vi "AlliGator Load Single Gate Image from PTU File.vi"(6 "Action":T1, 8 "error in (no error)":errorcluster, 10 "File Info":variant, 11 "Gate Index":i32) -> (0 "error out":errorcluster, 1 "Data 2":sgl[][](array[numeric]), 3 "Data 1":sgl[][](array[numeric]))   [LabVIEW 2021, in "AlliGator Files.lvlib"]
doc: "Loads single gate image from a .ptu file."
uses:
  AlliGator Files.lvlib
  HDF5/AlliGator FLI Image Stack Action.ctl
  PicoQuant/PTU/LabVIEW/Extended PicoQuant Data File Information.ctl
  PicoQuant/PTU/LabVIEW/PicoQuant Data File Information.ctl
  PicoQuant/PTU/LabVIEW/PicoQuant File Information.ctl
  PicoQuant/PTU/LabVIEW/PicoQuant Software Information.ctl
  PicoQuant/PTU/LabVIEW/PicoQuant Remote Request Information.ctl
  PicoQuant/PTU/LabVIEW/PicoQuant Hardware Information.ctl
  PicoQuant/PTU/LabVIEW/PicoQuant Input Channels.ctl
  PicoQuant/PTU/LabVIEW/PicoQuant Markers.ctl
  PicoQuant/PTU/LabVIEW/PicoQuant Modules.ctl
  PicoQuant/PTU/LabVIEW/PicoQuant Router Channels.ctl
  PicoQuant/PTU/LabVIEW/PicoQuant Measurement Information.ctl
  PicoQuant/PTU/LabVIEW/PicoQuant Image Information.ctl
  PicoQuant/PTU/LabVIEW/PicoQuant Results Format.ctl
  PicoQuant/PTU/LabVIEW/PicoQuant Measurement Results.ctl
  Globals, Variables, Constants/AlliGator Variables List.ctl
  PicoQuant/PTU/LabVIEW/Bin Photons in Pixels.vi
  PicoQuant/PTU/LabVIEW/Bin Nanotimes in Pixel.vi
  PicoQuant/PTU/LabVIEW/PTU Files.lvlib
  PicoQuant/PicoQuant.lvlib
  Globals, Variables, Constants/AlliGator Globals, Variables & Constants.lvlib
  Time/Time.lvlib
  HDF5/AlliGator HDF5.lvlib
panel:
  out "Time (s)":dbl
  # "see the AlliGator License on the block diagram (Ctrl+E or Window:Show Block Diagram)"
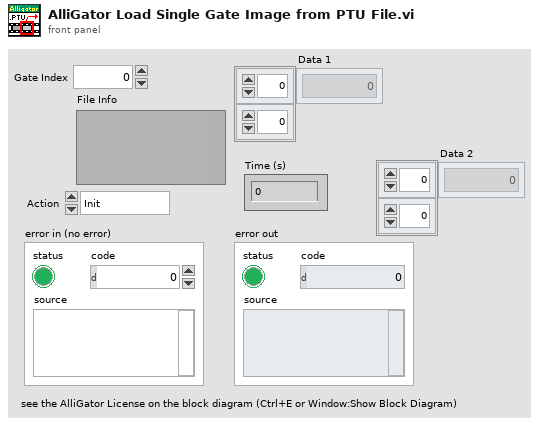
[diagram p1: front panel]
types:
  T1 = typedef "AlliGator HDF5.lvlib/AlliGator FLI Image Stack Action.ctl" = enum16{"Init", "Get Image", "Close"}
  T2 = typedef "PicoQuant.lvlib/Extended PicoQuant Data File Information.ctl" = cluster{"File Path":path, "Data offset (in bytes)":i64, "PicoQuant Data File Information":T3, "User defined # Gates":i64, "User defined Bin Size (s)":dbl, "p (# native bins per user bin)":dbl}
  T3 = typedef "PTU Files.lvlib/PicoQuant Data File Information.ctl" = cluster{"PQ File Information":T4, "PQ Software Information":T5, "PQ Remote Request Information":T6, "PQ Hardware Information":T7, "PQ Measurement Information":T12, "PQ Image Information":T13, "PQ TT Results Format Information":T14, "PQ Measurement Results":T15}
  T4 = typedef "PTU Files.lvlib/PicoQuant File Information.ctl" = cluster{"GUID":string, "Assured Content":string, "Measurement Mode":i64, "Measurement SubMode":i64, "Comment":string, "Creation Time":string}
  T5 = typedef "PTU Files.lvlib/PicoQuant Software Information.ctl" = cluster{"Content Version":string, "Name":string, "Version":string, "# Modules":i64, "Module Names":string[], "Module Versions":string[], "SVN Build":i64}
  T6 = typedef "PTU Files.lvlib/PicoQuant Remote Request Information.ctl" = cluster{"Started by Remote Interface":bool, "Measurement Type":i64, "# Pixel X":i64, "# Pixel Y":i64, "Record Version":i64, "Scanning Pattern":i64, "Scanning Resolution (m/px)":dbl, "Comment":string, "File Name":string, "Group Name":string}
  T7 = typedef "PTU Files.lvlib/PicoQuant Hardware Information.ctl" = cluster{"Input Channels":T8, "Markers":T9, "Modules":T10, "Router Channels":T11}
  T8 = typedef "PTU Files.lvlib/PicoQuant Input Channels.ctl" = cluster{"# Input Channels":i64, "CFD Levels (mV)":i64[], "CFD Zero Crossings (mV)":i64[], "CFD Channel Enabled":bool[], "Module Indices":i64[], "Offsets (ps)":i64[], "Td Codes":i64[], "Trigger Edges":i64[], "Trigger Levels (mV)":i64[]}
  T9 = typedef "PTU Files.lvlib/PicoQuant Markers.ctl" = cluster{"# Markers":i64, "Markers Enabled":bool[], "Holdoff (ns)":i64, "Rising Edges":bool[]}
  T10 = typedef "PTU Files.lvlib/PicoQuant Modules.ctl" = cluster{"# Modules":i64, "Type Codes":i64[], "Version Codes":i64[]}
  T11 = typedef "PTU Files.lvlib/PicoQuant Router Channels.ctl" = cluster{"# Router Channels":i64, "CFD Levels (mV)":i64[], "CFD Present":bool[], "CFD Zero Crossings (mV)":i64[], "Input Levels (mV)":i64[], "Input Types":i64[], "Offsets (ps)":i64[], "Rising Edges":bool[], "Router Enabled":bool, "Router Model Code":i64, "Router Version":string, "Sync CFD Level (mV)":i64, "Sync CFD Zero Crossing (mV)":i64, "Sync Divider":i64, "Sync Offset (ps)":i64, "Sync Trigger Edge":i64, "Sync Trigger Level (mV)":i64, "Trigger Out On":bool, "Trigger Out Period (s)":dbl, "Base Resolution (s)":dbl, "External Devices":i64, "External Reference Clock":bool, "Features":u64, "Part Number":string, "Serial Number (string)":string, "Serial Number":i64, "Timing Mode":i64, "Hardware Type":string, "Hardware Version":string}
  T12 = typedef "PTU Files.lvlib/PicoQuant Measurement Information.ctl" = cluster{"Acquisition Time (ms)":i64, "Binning Factor":i64, "Global Resolution (s)":dbl, "Invalid Sync":bool, "Offset (ns)":u64, "# Curve Parameters":u64, "Devices":string[], "Names":string[], "Start Values":dbl[], "Steps":dbl[], "Stop Values":dbl[], "Tag Names":string[], "Units":string[], "Resolution (s)":dbl, "Restart":bool, "Stop At":u64, "Stop on Over f1":bool}
  T13 = typedef "PTU Files.lvlib/PicoQuant Image Information.ctl" = cluster{"Hardware Acceleration":i64, "Bidirectional":bool, "Dimensions":i64, "Frame Marker":i64, "Scanner Identity":i64, "Learning Time (s)":i64, "Line Frequency":dbl, "Line Start Marker":i64, "Line Stop Marker":i64, "Max Frames":i64, "Objective Name":string, "Pixel Resolution (um)":dbl, "# Pixels X":i64, "# Pixels Y":i64, "Preview Pixels/Line":i64, "Scan Direction":i64, "Sinusoidal Correction":i64, "Time per Line (ms)":dbl, "Time per Pixel (ms)":i64, "Velocity":i64, "X0 (um)":dbl, "X1 (um)":dbl, "X Calibration Offset (V)":dbl, "X Calibration (m/V)":dbl, "Y0 (um)":dbl, "Y1 (um)":dbl, "Y Calibration Offset (V)":dbl, "Y Calibration (m/V)":dbl, "Z0 (um)":dbl, "Z1 (um)":dbl, "Z Calibration Offset (V)":dbl, "Z  Calibration (m/V)":dbl}
  T14 = typedef "PTU Files.lvlib/PicoQuant Results Format.ctl" = cluster{"Bits per Record":i64, "Channel Mask":i64, "Channel Shift ":i64, "DTime Mask":i64, "DTime Shift":i64, "Marker Mask":i64, "Marker Shift":i64, "NSync Mask":i64, "NSync Shift":i64, "Special Mask":i64, "TTTR Record Type":i64, "Wrap Around":i64}
  T15 = typedef "PTU Files.lvlib/PicoQuant Measurement Results.ctl" = cluster{"Stop Reason":i64, "Input Rates (cps)":i64[], "Warning Flags":u64, "# Records":i64, "Stop After (ms)":i64, "Sync Rate (cps)":i64}
  T16 = typedef "AlliGator Globals, Variables & Constants.lvlib/AlliGator Variables List.ctl" = enum16{"---- GUI ----", "GUI:Initialization Status", "GUI:State Indicators Refnum", "GUI:Original AlliGator Menu Items", "GUI:Current Action Loop State", "GUI:Script in progress", "GUI:Playback", "GUI:Loop Playback", "GUI:Search ROI Used", "GUI:Search ROI", "Decay Graph Max Legend Size", "Intensity Graph Max Legend Size", "Decay Statistics Graph Max Legend Size", "Phasor Graph Max Legend Size", "Phasor Ratio Graph Max Legend Size", "Lifetime Graph Max Legend Size", "---- Files ----", "Files:Export Dataset Frames as Individual Files", "Files:Show Batch Export Help Balloons", "Files:Frames in Dataset", "Files:ptu File Frame Start Indices", "Files:Current Frame in Dataset", "Files:Current Frame Timestamp", "Files:Dataset Loaded", "Files:Dataset Metadata", "Files:Dataset Channel", "Files:Dataset Data Description", "Files:Background Dataset Metadata", "Files:Background Dataset Channel", "Files:Background Dataset Data Description", "Files:Background File Subtraction", "Files:Background File Path", "Files:Background File Pile-up Correction", "Files:Background File Pixel Well Capacity", "Files:Background File Scaling Factor", "Files:Current Dataset Load Settings", "Files:Dataset Path", "Files:ICCD-specific Information", "Files:Macrotime Gate Separation", "------ Python Plugins ------", "Python Plugins:Information", "Python Plugins:Python Session", "Python Plugins:Valid Python Session?", "---- Source Image ----", "Source Image:ROIs", "Source Image:Current ROI", "Source Image:ROI Event Refnum", "X_Source Image Display Range", "X_Source Image Palette Information", "X_Type of Displayed Image", "X_Time Gate Slider", "Source Image:Palette List", "Source Image:Scale", "Source Image:ROI Overlay Color", "Source Image:Overlay to Erase", "Source Image:Is Displayed Image Accumulated", "Source Image:White Light Image Modified", "Source Image:Mask Image Modified", "---- Image Profile Window ----", "Image Profile:Window Event Refnum", "Image Profile:IntensityType", "Image Profile:Intensity Average Type", "Image Profile:Intensity-weighted SDV", "Image Profile:Box Profile Type", "Image Profile:Window Open", "Image Profile:Plotted Fit Parameter", "------ Phasor Graph -------", "Phasor Graph:Show Line", "---- Phasor Plot ---", "Phasor Plot:Parameters Changed", "Phasor Plot:FLI Dataset Modified since last Calculation", "Phasor Harmonics Data", "Selected Phasor Harmonics", "Phasor Harmonic Manager Event Refnum", "Phasor Plot:ROIs", "Phasor Plot:Current ROI", "Phasor Plot:ROI Event Refnum", "Phasor Plot:Image Reference Points", "Phasor Plot:Computed", "Phasor Plot:Palette Information", "Phasor Plot:Palette List", "Phasor Plot:Phasor Ratio Palette Information", "Phasor Plot:Phasor Ratio Palette List", "Phasor Plot:Image Scale", "Phasor Plot:Image Overlay to Erase", "Phasor Plot:Image Elements to Update", "Phasor Plot:Current Calculation Parameters", "Phasor Plot:Current Calibration Options", "Phasor Plot:Reset Cumulated Phasor Plot", "Phasor Plot:Reference 1", "Phasor Plot:Lifetime Reference 1", "Phasor Plot:Reference 1 Frequency", "Phasor Plot:Reference 2", "Phasor Plot:Lifetime Reference 2", "Phasor Plot:Reference 2 Frequency", "---- Decay Analysis ----", "Number of Selected Decays to Fit", "LS Fit Results", "LAR Fit Results", "BS Fit Results", "Last Decay Max - Min", "Best Fit Parameters", "Best Fit Parameter Names", "Actual Size X", "Actual Size Y", "Binning X", "Binning Y", "Actual # Gates", "Dataset Number", "Gates to...", "Gates Skipped", "Gates to keep", "Gate Step", "Gate Separation", "Reversed Gates", "Pile-up Correction", "Pixel Well Capacity", "Background Subtracted", "Background Subtraction Method", "Background Definition Range", "Background File (deprecated)", "Number of Dataset Accumulated", "Array of Accumulated Dataset Paths", "Do Averaged Datasets", "Destination File Path", "Process Plot Target", "Use 1/D as Phasor Frequency", "---- Decay Fit Parameter Map -----", "Decay Fit Parameter Map:Palette Information", "Decay Fit Parameter Map:Palette List", "---- Parameter Map ----", "Parameter Map:Palette Information", "Parameter Map:Palette List", "------- Local Decay Window ---------", "Local Decay Graph Window:Event Refnum", "Local Decay Graph Window:Use normalized IRF for convolution", "----- Miscellaneous ----", "Misc:Skippable Dialog Windows Status"}
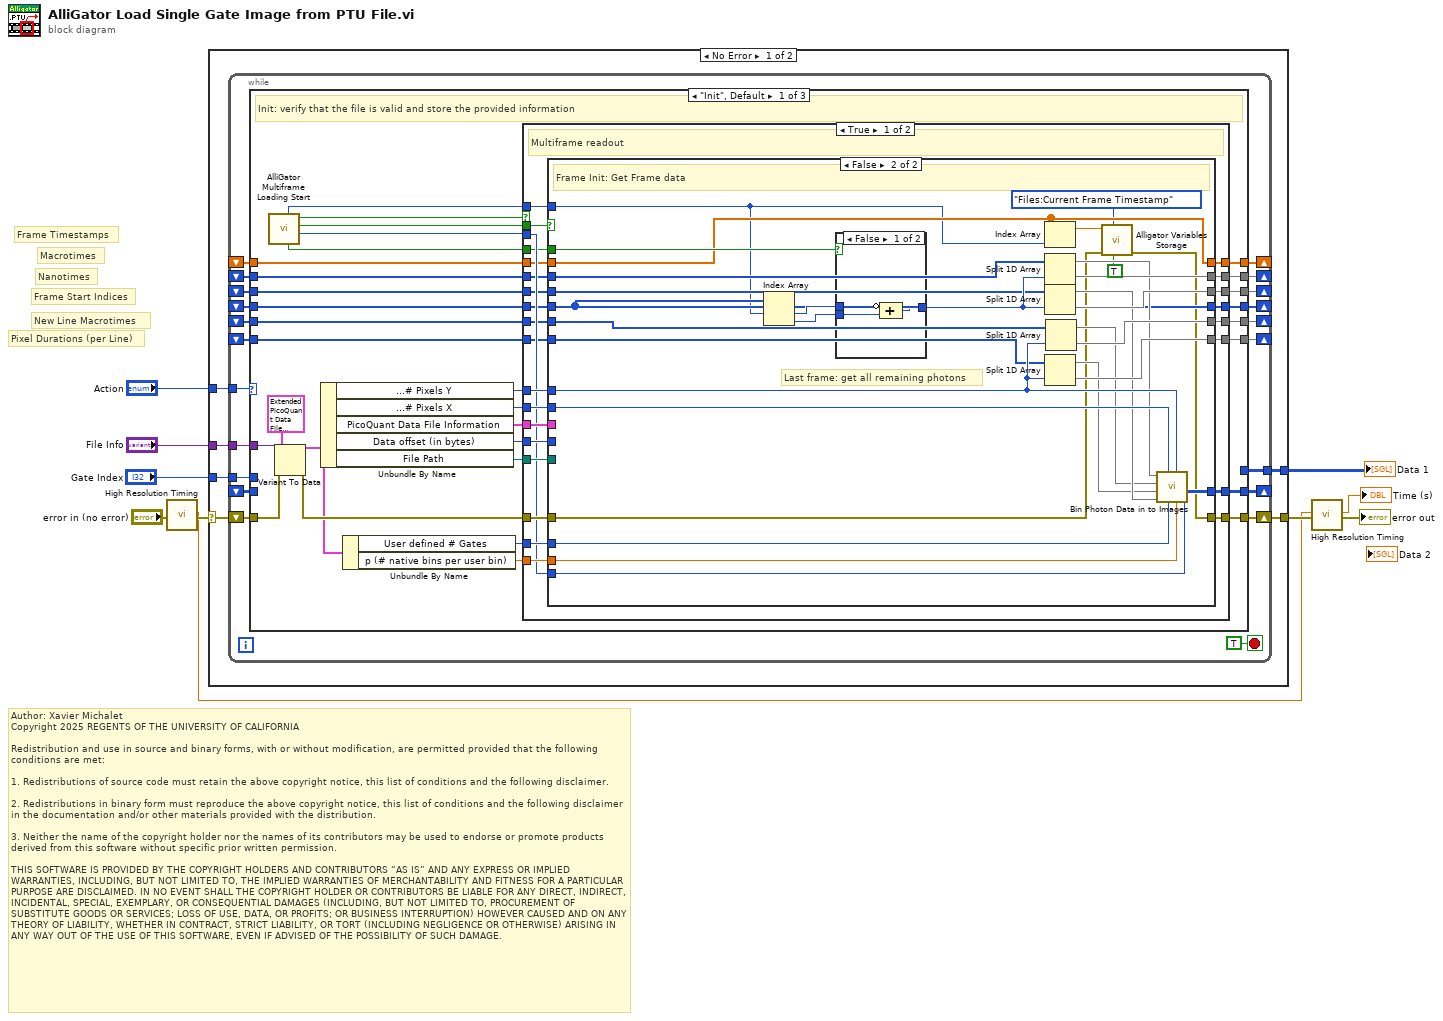
[diagram p0: block diagram]
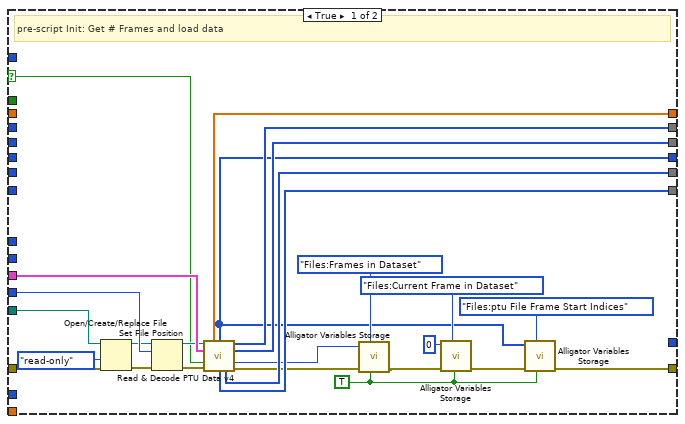
[diagram p2: hidden frame]
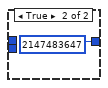
[diagram p3: hidden frame]
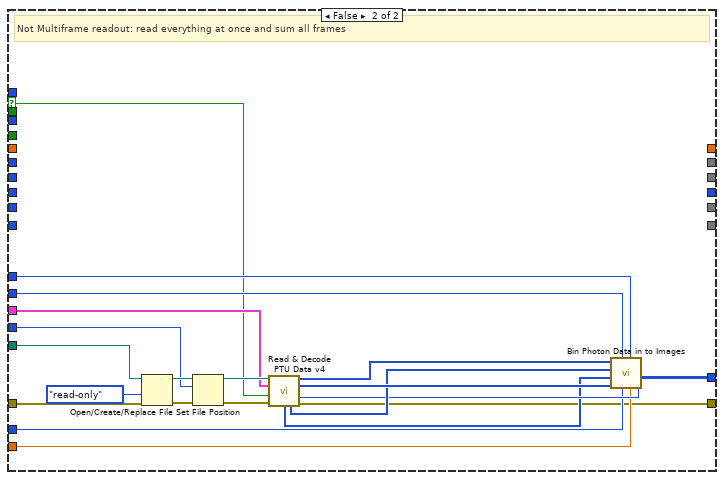
[diagram p4: hidden frame]
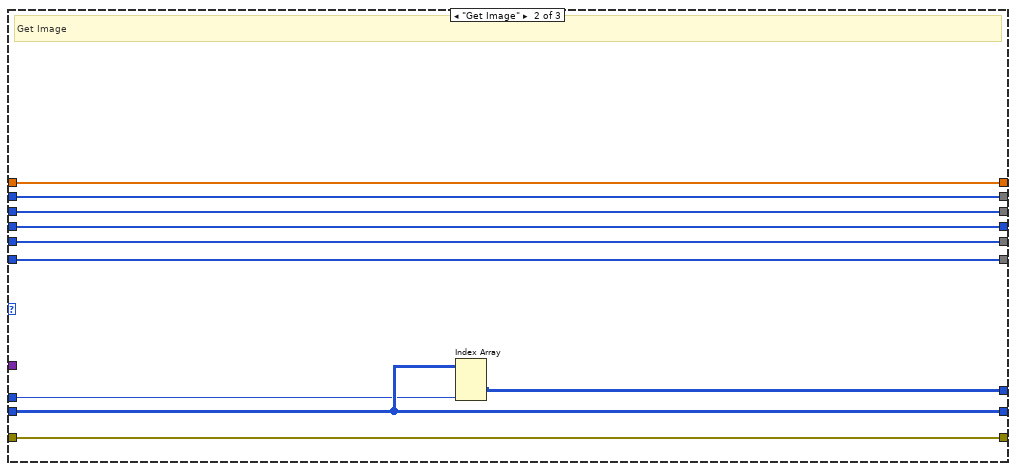
[diagram p5: hidden frame]
diagram:
  # "Author: Xavier Michalet\nCopyright 2025 REGENTS OF THE UNIVERSITY OF CALIFORNIA\n\nRedistribution and use in source and binary forms, with or without modification, are permitted provided that the following conditions are met:\n\n1. Redistributions of source code must retain the above copyright notice, this list of conditions and the following disclaimer.\n\n2. Redistributions in binary form must reproduce the above copyright notice, this list of conditions and the following disclaimer in the documentation and/or other materials provided with the distribution.\n\n3. Neither the name of the copyright holder nor the names of its contributors may be used to endorse or promote products derived from this software without specific prior written permission.\n\nTHIS SOFTWARE IS PROVIDED BY THE COPYRIGHT HOLDERS AND CONTRIBUTORS “AS IS” AND ANY EXPRESS OR IMPLIED WARRANTIES, INCLUDING, BUT NOT LIMITED TO, THE IMPLIED WARRANTIES OF MERCHANTABILITY AND FITNESS FOR A PARTICULAR PURPOSE ARE DISCLAIMED. IN NO EVENT SHALL THE COPYRIGHT HOLDER OR CONTRIBUTORS BE LIABLE FOR ANY DIRECT, INDIRECT, INCIDENTAL, SPECIAL, EXEMPLARY, OR CONSEQUENTIAL DAMAGES (INCLUDING, BUT NOT LIMITED TO, PROCUREMENT OF SUBSTITUTE GOODS OR SERVICES; LOSS OF USE, DATA, OR PROFITS; OR BUSINESS INTERRUPTION) HOWEVER CAUSED AND ON ANY THEORY OF LIABILITY, WHETHER IN CONTRACT, STRICT LIABILITY, OR TORT (INCLUDING NEGLIGENCE OR OTHERWISE) ARISING IN ANY WAY OUT OF THE USE OF THIS SOFTWARE, EVEN IF ADVISED OF THE POSSIBILITY OF SUCH DAMAGE."
  # "Frame Timestamps"
  # "Pixel Durations (per Line)"
  # "New Line Macrotimes"
  # "Nanotimes"
  # "Macrotimes"
  # "Frame Start Indices"
  n1 = call "High Resolution Timing.vi"("Error In"="error in (no error)") -> ("elapsed (relative) seconds"=w2:dbl, "Error Out"=w4:errorcluster)  [unwired: 16 in, 1 out]
  n2 = case shown="No Error" w4 {
    selector: w4 -> [w15 w193]
    tunnel: [w14 w193] -> w9
    tunnel: "Action" -> [w16 _]
    tunnel: "File Info" -> [w13 _]
    tunnel: "Gate Index" -> [w12 _]
    tunnel: [w11 _] -> w5
    frame No Error {
      n3 = while {
        tunnel: w16 -> [w36]
        tunnel: w13 -> [w33]
        tunnel: w12 -> [w32]
        tunnel: [w31] -> w11
        shift-right: [w30] -> _
        shift-left: _ -> [w29]
        shift-right: [w34] -> w14
        shift-left: w15 -> [w35]
        shift-right: [w28] -> _
        shift-left: _ -> [w25]
        shift-right: [w27] -> _
        shift-left: _ -> [w24]
        shift-right: [w26] -> _
        shift-left: _ -> [w23]
        shift-right: [w22] -> _
        shift-left: _ -> [w20]
        shift-right: [w21] -> _
        shift-left: _ -> [w19]
        shift-right: [w18] -> _
        shift-left: _ -> [w17]
        stop <- TRUE stop-if-true
        n4 = case shown="\"Init\", Default" w36 {
          tunnel: w35 -> [w67 w185 w192]
          tunnel: [w40 w185 w192] -> w34
          tunnel: w33 -> [w68 _ _]
          tunnel: w32 -> [_ w183 _]
          tunnel: [_ w182 _] -> w31
          tunnel: [w63 w184 _] -> w30
          tunnel: w29 -> [_ w184 _]
          tunnel: [w62 w181 w191] -> w28
          tunnel: [w61 w180 w190] -> w27
          tunnel: [w60 w179 w189] -> w26
          tunnel: w25 -> [w50 w181 w191]
          tunnel: w24 -> [w49 w180 w190]
          tunnel: w23 -> [w48 w179 w189]
          tunnel: [w47 w178 w188] -> w22
          tunnel: [w46 w177 w187] -> w21
          tunnel: w20 -> [w45 w178 w188]
          tunnel: w19 -> [w44 w177 w187]
          tunnel: [w39 w176 w186] -> w18
          tunnel: w17 -> [w38 w176 w186]
          frame "Init", Default {
            # "Init: verify that the file is valid and store the provided information"
            n5 = call "AlliGator Multiframe Loading Start.vi"() -> ("# Frames"=w43:i32, "Multiframe Start?"=w51:bool, "Multiframe?"=w52:bool, "Last Frame?"=w41:bool, "Current Frame Index"=w42:i32)  [unwired: 6 in, 1 out]
            n6 = Variant To Data(error in=w67, type=T2 {"File Path"=path "", "Data offset (in bytes)"=0, "PicoQuant Data File Information"={"PQ File Information"={"GUID"="", "Assured Content"="", "Measurement Mode"=0, "Measurement SubMode"=0, "Comment"="", "Creation Time"=""}, "PQ Software Information"={"Content Version"="", "Name"="", "Version"="", "# Modules"=0, "Module Names"=[], "Module Versions"=[], "SVN Build"=0}, "PQ Remote Request Information"={"Started by Remote Interface"=FALSE, "Measurement Type"=0, "# Pixel X"=0, "# Pixel Y"=0, "Record Version"=0, "Scanning Pattern"=0, "Scanning Resolution (m/px)"=0.0, "Comment"="", "File Name"="", "Group Name"=""}, "PQ Hardware Information"={"Input Channels"={"# Input Channels"=0, "CFD Levels (mV)"=[], "CFD Zero Crossings (mV)"=[], "CFD Channel Enabled"=[], "Module Indices"=[], "Offsets (ps)"=[], "Td Codes"=[], "Trigger Edges"=[], "Trigger Levels (mV)"=[]}, "Markers"={"# Markers"=0, "Markers Enabled"=[], "Holdoff (ns)"=0, "Rising Edges"=[]}, "Modules"={"# Modules"=0, "Type Codes"=[], "Version Codes"=[]}, "Router Channels"={"# Router Channels"=0, "CFD Levels (mV)"=[], "CFD Present"=[], "CFD Zero Crossings (mV)"=[], "Input Levels (mV)"=[], "Input Types"=[], "Offsets (ps)"=[], "Rising Edges"=[], "Router Enabled"=FALSE, "Router Model Code"=0, "Router Version"="", "Sync CFD Level (mV)"=0, "Sync CFD Zero Crossing (mV)"=0, "Sync Divider"=0, "Sync Offset (ps)"=0, "Sync Trigger Edge"=0, "Sync Trigger Level (mV)"=0, "Trigger Out On"=FALSE, "Trigger Out Period (s)"=0.0, "Base Resolution (s)"=0.0, "External Devices"=0, "External Reference Clock"=FALSE, "Features"=0, "Part Number"="", "Serial Number (string)"="", "Serial Number"=0, "Timing Mode"=0, "Hardware Type"="", "Hardware Version"=""}}, "PQ Measurement Information"={"Acquisition Time (ms)"=0, "Binning Factor"=0, "Global Resolution (s)"=0.0, "Invalid Sync"=FALSE, "Offset (ns)"=0, "# Curve Parameters"=0, "Devices"=[], "Names"=[], "Start Values"=[], "Steps"=[], "Stop Values"=[], "Tag Names"=[], "Units"=[], "Resolution (s)"=0.0, "Restart"=FALSE, "Stop At"=0, "Stop on Over f1"=FALSE}, "PQ Image Information"={"Hardware Acceleration"=0, "Bidirectional"=FALSE, "Dimensions"=0, "Frame Marker"=0, "Scanner Identity"=0, "Learning Time (s)"=0, "Line Frequency"=0.0, "Line Start Marker"=0, "Line Stop Marker"=0, "Max Frames"=0, "Objective Name"="", "Pixel Resolution (um)"=0.0, "# Pixels X"=0, "# Pixels Y"=0, "Preview Pixels/Line"=0, "Scan Direction"=0, "Sinusoidal Correction"=0, "Time per Line (ms)"=0.0, "Time per Pixel (ms)"=0, "Velocity"=0, "X0 (um)"=0.0, "X1 (um)"=0.0, "X Calibration Offset (V)"=0.0, "X Calibration (m/V)"=0.0, "Y0 (um)"=0.0, "Y1 (um)"=0.0, "Y Calibration Offset (V)"=0.0, "Y Calibration (m/V)"=0.0, "Z0 (um)"=0.0, "Z1 (um)"=0.0, "Z Calibration Offset (V)"=0.0, "Z  Calibration (m/V)"=0.0}, "PQ TT Results Format Information"={"Bits per Record"=0, "Channel Mask"=0, "Channel Shift "=0, "DTime Mask"=0, "DTime Shift"=0, "Marker Mask"=0, "Marker Shift"=0, "NSync Mask"=0, "NSync Shift"=0, "Special Mask"=0, "TTTR Record Type"=0, "Wrap Around"=0}, "PQ Measurement Results"={"Stop Reason"=0, "Input Rates (cps)"=[], "Warning Flags"=0, "# Records"=0, "Stop After (ms)"=0, "Sync Rate (cps)"=0}}, "User defined # Gates"=0, "User defined Bin Size (s)"=0.0, "p (# native bins per user bin)"=0.0} ("Extended PicoQuant Data File Information"), Variant=w68) -> (data=w64:T2, error out=w66:errorcluster)
            n7 = Unbundle By Name(w64) -> ("PicoQuant Data File Information.PQ Image Information.# Pixels Y"=w57:i64, "PicoQuant Data File Information.PQ Image Information.# Pixels X"=w56:i64, "PicoQuant Data File Information"=w55:T3, "Data offset (in bytes)"=w59:i64, "File Path"=w58:path)
            n8 = Unbundle By Name(w64) -> ("User defined # Gates"=w54:i64, "p (# native bins per user bin)"=w53:dbl)
            n9 = case shown="True" w52 {
              selector: w52 -> [_ w155]
              tunnel: w66 -> [w94 w175]
              tunnel: [w93 w174] -> w63
              tunnel: [w86 _] -> w62
              tunnel: [w85 _] -> w61
              tunnel: [w81 _] -> w60
              tunnel: w59 -> [w92 w164]
              tunnel: w58 -> [w91 w162]
              tunnel: w57 -> [w84 w161]
              tunnel: w56 -> [w90 w160]
              tunnel: w55 -> [w89 w159]
              tunnel: w54 -> [w88 w158]
              tunnel: w53 -> [w87 w157]
              tunnel: w51 -> [w77 _]
              tunnel: w50 -> [w76 _]
              tunnel: w49 -> [w75 _]
              tunnel: w48 -> [w74 _]
              tunnel: [w83 _] -> w47
              tunnel: [w82 _] -> w46
              tunnel: w43 -> [w80 _]
              tunnel: w45 -> [w73 _]
              tunnel: w44 -> [w72 _]
              tunnel: w42 -> [w79 _]
              tunnel: w41 -> [w78 _]
              tunnel: [w71 w156] -> w40
              tunnel: [w70 _] -> w39
              tunnel: w38 -> [w69 _]
              frame True {
                # "Multiframe readout"
                n10 = case shown="False" w77 {
                  selector: w77 -> [w96 _]
                  tunnel: w94 -> [w120 w122]
                  tunnel: [_ w150] -> w93
                  tunnel: w92 -> [w119 _]
                  tunnel: w91 -> [w118 _]
                  tunnel: w90 -> [_ w149]
                  tunnel: w89 -> [w117 _]
                  tunnel: w88 -> [_ w148]
                  tunnel: w87 -> [_ w147]
                  tunnel: [w111 w146] -> w86
                  tunnel: [w110 w145] -> w85
                  tunnel: w84 -> [_ w144]
                  tunnel: [w109 w143] -> w83
                  tunnel: [w108 w142] -> w82
                  tunnel: [w97 w130] -> w81
                  tunnel: w80 -> [_ w141]
                  tunnel: w79 -> [_ w126]
                  tunnel: w78 -> [_ w140]
                  tunnel: w76 -> [_ w132]
                  tunnel: w75 -> [_ w131]
                  tunnel: w74 -> [_ w130]
                  tunnel: w73 -> [_ w129]
                  tunnel: w72 -> [_ w128]
                  tunnel: [w100 w121] -> w71
                  tunnel: [w95 w127] -> w70
                  tunnel: w69 -> [_ w127]
                  frame True {
                    w99 = TRUE ("Get(F)/Set")
                    # "pre-script Init: Get # Frames and load data"
                    n11 = Open/Create/Replace File(file path (use dialog)=w118, error in=w120, access (0:read/write)=enum16{"read/write", "read-only", "write-only"}."read-only") -> (refnum out=w113:refnum<file>, error out=w116:errorcluster)  [unwired: 3 in, 1 out]
                    n12 = Set File Position(offset (in bytes) (0)=w119, refnum=w113, error in=w116) -> (refnum out=w112:refnum<file>, error out=w114:errorcluster)  [unwired: 1 in]
                    n13 = call "Read & Decode PTU Data v4.vi"("Byte Stream File in"=w112, "PicoQuant Data File Information"=w117, "Multiframe Readout"=w96, "error in (no error)"=w114) -> ("Frame Timestamps (s)"=w95:dbl[], "Frame Start Indices"=w97:i32[], "Macrotimes"=w111:u64[], "Nanotimes"=w110:u32[], "# Frames (inferred)"=w105:i32, "Pixel Durations (inferred_"=w108:i64[], "Line Start Macrotimes"=w109:u64[], "Error Out"=w107:errorcluster)  [unwired: 2 in, 2 out]
                    n14 = call "Alligator Variables Storage.vi"("Get(F)/Set"=w99, "AlliGator Variable"=AlliGator_Variables_List."Files:Frames in Dataset" ("Alligator Variable"), "Error In"=w107, "Data in"=w105) -> ("Error Out"=w104:errorcluster)  [unwired: 5 in, 2 out]
                    n15 = call "Alligator Variables Storage.vi"("Get(F)/Set"=w99, "AlliGator Variable"=AlliGator_Variables_List."Files:Current Frame in Dataset" ("Alligator Variable"), "Error In"=w104, "Data in"=0 ("# Frames")) -> ("Error Out"=w101:errorcluster)  [unwired: 5 in, 2 out]
                    n16 = call "Alligator Variables Storage.vi"("Get(F)/Set"=w99, "AlliGator Variable"=AlliGator_Variables_List."Files:ptu File Frame Start Indices" ("Alligator Variable"), "Error In"=w101, "Data in"=w97) -> ("Error Out"=w100:errorcluster)  [unwired: 5 in, 2 out]
                  }
                  frame False {
                    # "Last frame: get all remaining photons"
                    # "Frame Init: Get Frame data"
                    n17 = Index Array(array=w130, index #1=w126) -> (element #1=w135:i32, element #2=w134:i32)  [unwired: 1 in]
                    n18 = case shown="False" w140 {
                      tunnel: w135 -> [w153 _]
                      tunnel: w134 -> [w152 _]
                      tunnel: [w151 2147483647] -> w133
                      frame False {
                        n19 = Compound Arithmetic op=ADD(invert w153, w152) -> (w151:i32)
                      }
                      frame True {
                      }
                    }
                    n20 = Index Array(array=w127, index=w126) -> (element=w125:dbl)
                    n21 = Split 1D Array(array=w132, index=w133) -> (first subarray=w139:u64[], second subarray=w146:u64[])
                    n22 = Split 1D Array(array=w131, index=w133) -> (first subarray=w138:u32[], second subarray=w145:u32[])
                    n23 = Split 1D Array(array=w128, index=w144) -> (first subarray=w136:i64[], second subarray=w142:i64[])
                    n24 = Split 1D Array(array=w129, index=w144) -> (first subarray=w137:u64[], second subarray=w143:u64[])
                    n25 = call "Alligator Variables Storage.vi"("Get(F)/Set"=TRUE, "AlliGator Variable"=AlliGator_Variables_List."Files:Current Frame Timestamp" ("Alligator Variable"), "Error In"=w122, "Data in"=w125) -> ("Error Out"=w121:errorcluster)  [unwired: 5 in, 2 out]
                    n26 = call "Bin Photon Data in to Images.vi"("# Frames"=w141, "# native bins per user bin (Gate Step/Bin Width)"=w147, "# Pixels Y"=w144, "# Gates"=w148, "# Pixels X"=w149, "Nanotimes"=w138, "Pixel Durations"=w136, "New Line Macrotimes"=w137, "Macrotimes"=w139) -> ("Gate Images"=w150:u16[][][])  [unwired: 1 in, 1 out]
                  }
                }
              }
              frame False {
                # "Not Multiframe readout: read everything at once and sum all frames"
                n27 = Open/Create/Replace File(file path (use dialog)=w162, error in=w175, access (0:read/write)=enum16{"read/write", "read-only", "write-only"}."read-only") -> (refnum out=w166:refnum<file>, error out=w169:errorcluster)  [unwired: 3 in, 1 out]
                n28 = Set File Position(offset (in bytes) (0)=w164, refnum=w166, error in=w169) -> (refnum out=w165:refnum<file>, error out=w167:errorcluster)  [unwired: 1 in]
                n29 = call "Read & Decode PTU Data v4.vi"("Byte Stream File in"=w165, "PicoQuant Data File Information"=w159, "Multiframe Readout"=w155, "error in (no error)"=w167) -> ("Macrotimes"=w173:u64[], "Nanotimes"=w172:u32[], "# Frames (inferred)"=w170:i32, "Pixel Durations (inferred_"=w163:i64[], "Line Start Macrotimes"=w171:u64[], "Error Out"=w156:errorcluster)  [unwired: 2 in, 4 out]
                n30 = call "Bin Photon Data in to Images.vi"("# Frames"=w170, "# native bins per user bin (Gate Step/Bin Width)"=w157, "# Pixels Y"=w161, "# Gates"=w158, "# Pixels X"=w160, "Nanotimes"=w172, "Pixel Durations"=w163, "New Line Macrotimes"=w171, "Macrotimes"=w173) -> ("Gate Images"=w174:u16[][][])  [unwired: 1 in, 1 out]
              }
            }
          }
          frame "Get Image" {
            # "Get Image"
            n31 = Index Array(array=w184, index (dim 2)=w183) -> (element=w182:u16[][])  [unwired: 2 in]
          }
          frame "Close" {
            # "Close File"
          }
        }
      }
    }
    frame Error {
    }
  }
  "Data 1" <- w5
  n32 = call "High Resolution Timing.vi"("relative seconds (NaN)"=w2, "Error In"=w9) -> ("elapsed (relative) seconds"=→"Time (s)":dbl, "Error Out"=→"error out":errorcluster)  [unwired: 15 in, 1 out]
